vi "Send.vi"(10 "Error":errorcluster) -> (3 "Error Msg Strategy out":refnum<class "Error Msg Strategy.lvclass">)   [LabVIEW 2021, in "Error.lvlib" / "Error Msg Strategy.lvclass"]
uses:
  Error Msg Strategy.lvclass
  Error Msg Strategy.lvclass/Error Msg Strategy.ctl
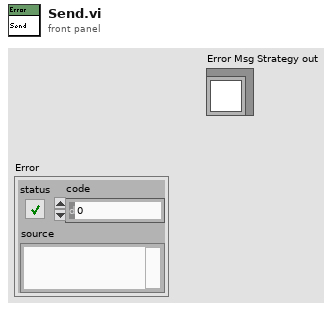
[diagram p1: front panel]
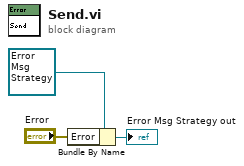
[diagram p0: block diagram]
diagram:
  n1 = Bundle By Name(cluster=refnum<class "Error Msg Strategy.lvclass"> refnum ("Error Msg Strategy out"), "Error"="Error") -> (→"Error Msg Strategy out":refnum<class "Error Msg Strategy.lvclass">)
